vi "test_RS-xxx Protocol Factory.vi"(8 "error in (no error)":errorcluster, 11 "TestCase in":refnum<class "Instrument Addon Scripting API Protocol Factories Unit Tests.lvclass">) -> (0 "error out":errorcluster, 3 "TestCase out":refnum<class "Instrument Addon Scripting API Protocol Factories Unit Tests.lvclass">)   [LabVIEW 2018, in "Instrument Addon Scripting API Protocol Factories Unit Tests.lvclass"]
uses:
  Instrument Addon Scripting API Protocol Factories Unit Tests.lvclass
  RS-xxx/RS-xxx Settings.ctl
  RS-xxx/RS-xxx.lvclass
  RS-xxx/RS-xxx.lvclass/RS-xxx.ctl
  RS-xxx/Data Access/Read PortSettings.vi
  <vilib>/addons/_JKI Toolkits/VI Tester/TestCase.llb/TestCase.lvclass
  C:/Program Files (x86)/National Instruments/LabVIEW 2018/vi.lib/addons/_JKI Toolkits/VI Tester/TestCase.llb/TestCase.lvclass
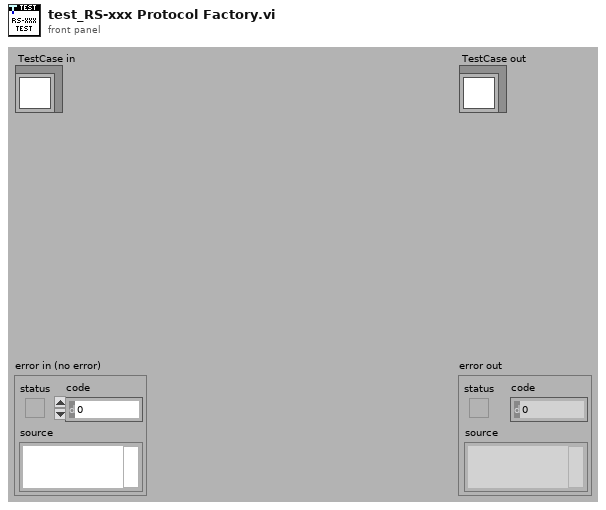
[diagram p1: front panel]
types:
  T1 = typedef "Protocols.lvlib/RS-xxx.lvclass/RS-xxx Settings.ctl" = cluster{"Port":string, "Baud Rate":u32, "Data Bits":u16, "Parity":enum16{"None", "Odd", "Even", "Mark", "Space"}, "Stop Bits":u16, "Flow Control":u16, "XON":enum16{"NUL", "SOH", "STX", "ETX", "EOT", "ENQ", "ACK", "BEL", "BS", "HT", "LF", "VT", "FF", "CR", "SO", "SI", "DLE", "DC1", "DC2", "DC3", "DC4", "NAK", "SYN", "ETB", "CAN", "EM", "SUB", "ESC", "FS", "GS", "RS", "US", "SP", "!", "\"", "#", "$", "%", "&", "'", "(", ")", "*", "+", ",", "- (-)", ".", "/", "0", "1", "2", "3", "4", "5", "6", "7", "8", "9", ":", ";", "<", "=", ">", "?", "@", "A", "B", "C", "D", "E", "F", "G", "H", "I", "J", "K", "L", "M", "N", "O", "P", "Q", "R", "S", "T", "U", "V", "W", "X", "Y", "Z", "[", "\\", "]", "^", "_", "`", "a", "b", "c", "d", "e", "f", "g", "h", "i", "j", "k", "l", "m", "n", "o", "p", "q", "r", "s", "t", "u", "v", "w", "x", "y", "z", "{", "|", "}", "~"}, "XOFF":enum16{"NUL", "SOH", "STX", "ETX", "EOT", "ENQ", "ACK", "BEL", "BS", "HT", "LF", "VT", "FF", "CR", "SO", "SI", "DLE", "DC1", "DC2", "DC3", "DC4", "NAK", "SYN", "ETB", "CAN", "EM", "SUB", "ESC", "FS", "GS", "RS", "US", "SP", "!", "\"", "#", "$", "%", "&", "'", "(", ")", "*", "+", ",", "- (-)", ".", "/", "0", "1", "2", "3", "4", "5", "6", "7", "8", "9", ":", ";", "<", "=", ">", "?", "@", "A", "B", "C", "D", "E", "F", "G", "H", "I", "J", "K", "L", "M", "N", "O", "P", "Q", "R", "S", "T", "U", "V", "W", "X", "Y", "Z", "[", "\\", "]", "^", "_", "`", "a", "b", "c", "d", "e", "f", "g", "h", "i", "j", "k", "l", "m", "n", "o", "p", "q", "r", "s", "t", "u", "v", "w", "x", "y", "z", "{", "|", "}", "~"}, "End Read on Termination Character":bool, "End Write on Termination Character":bool, "Termination Character":u8}
  T2 = cluster{"Port":string, "Baud Rate":u32, "Data Bits":u16, "Parity":enum16{"None", "Odd", "Even", "Mark", "Space"}, "Stop Bits":u16, "Flow Control":u16, "XON":enum16{"NUL", "SOH", "STX", "ETX", "EOT", "ENQ", "ACK", "BEL", "BS", "HT", "LF", "VT", "FF", "CR", "SO", "SI", "DLE", "DC1", "DC2", "DC3", "DC4", "NAK", "SYN", "ETB", "CAN", "EM", "SUB", "ESC", "FS", "GS", "RS", "US", "SP", "!", "\"", "#", "$", "%", "&", "'", "(", ")", "*", "+", ",", "- (-)", ".", "/", "0", "1", "2", "3", "4", "5", "6", "7", "8", "9", ":", ";", "<", "=", ">", "?", "@", "A", "B", "C", "D", "E", "F", "G", "H", "I", "J", "K", "L", "M", "N", "O", "P", "Q", "R", "S", "T", "U", "V", "W", "X", "Y", "Z", "[", "\\", "]", "^", "_", "`", "a", "b", "c", "d", "e", "f", "g", "h", "i", "j", "k", "l", "m", "n", "o", "p", "q", "r", "s", "t", "u", "v", "w", "x", "y", "z", "{", "|", "}", "~"}, "XOFF":enum16{"NUL", "SOH", "STX", "ETX", "EOT", "ENQ", "ACK", "BEL", "BS", "HT", "LF", "VT", "FF", "CR", "SO", "SI", "DLE", "DC1", "DC2", "DC3", "DC4", "NAK", "SYN", "ETB", "CAN", "EM", "SUB", "ESC", "FS", "GS", "RS", "US", "SP", "!", "\"", "#", "$", "%", "&", "'", "(", ")", "*", "+", ",", "- (-)", ".", "/", "0", "1", "2", "3", "4", "5", "6", "7", "8", "9", ":", ";", "<", "=", ">", "?", "@", "A", "B", "C", "D", "E", "F", "G", "H", "I", "J", "K", "L", "M", "N", "O", "P", "Q", "R", "S", "T", "U", "V", "W", "X", "Y", "Z", "[", "\\", "]", "^", "_", "`", "a", "b", "c", "d", "e", "f", "g", "h", "i", "j", "k", "l", "m", "n", "o", "p", "q", "r", "s", "t", "u", "v", "w", "x", "y", "z", "{", "|", "}", "~"}, "End Read on Termination Character":bool, "End Write on Termination Character":bool, "Termination Character":u8}
  T3 = enum16{"NUL", "SOH", "STX", "ETX", "EOT", "ENQ", "ACK", "BEL", "BS", "HT", "LF", "VT", "FF", "CR", "SO", "SI", "DLE", "DC1", "DC2", "DC3", "DC4", "NAK", "SYN", "ETB", "CAN", "EM", "SUB", "ESC", "FS", "GS", "RS", "US", "SP", "!", "\"", "#", "$", "%", "&", "'", "(", ")", "*", "+", ",", "- (-)", ".", "/", "0", "1", "2", "3", "4", "5", "6", "7", "8", "9", ":", ";", "<", "=", ">", "?", "@", "A", "B", "C", "D", "E", "F", "G", "H", "I", "J", "K", "L", "M", "N", "O", "P", "Q", "R", "S", "T", "U", "V", "W", "X", "Y", "Z", "[", "\\", "]", "^", "_", "`", "a", "b", "c", "d", "e", "f", "g", "h", "i", "j", "k", "l", "m", "n", "o", "p", "q", "r", "s", "t", "u", "v", "w", "x", "y", "z", "{", "|", "}", "~"}
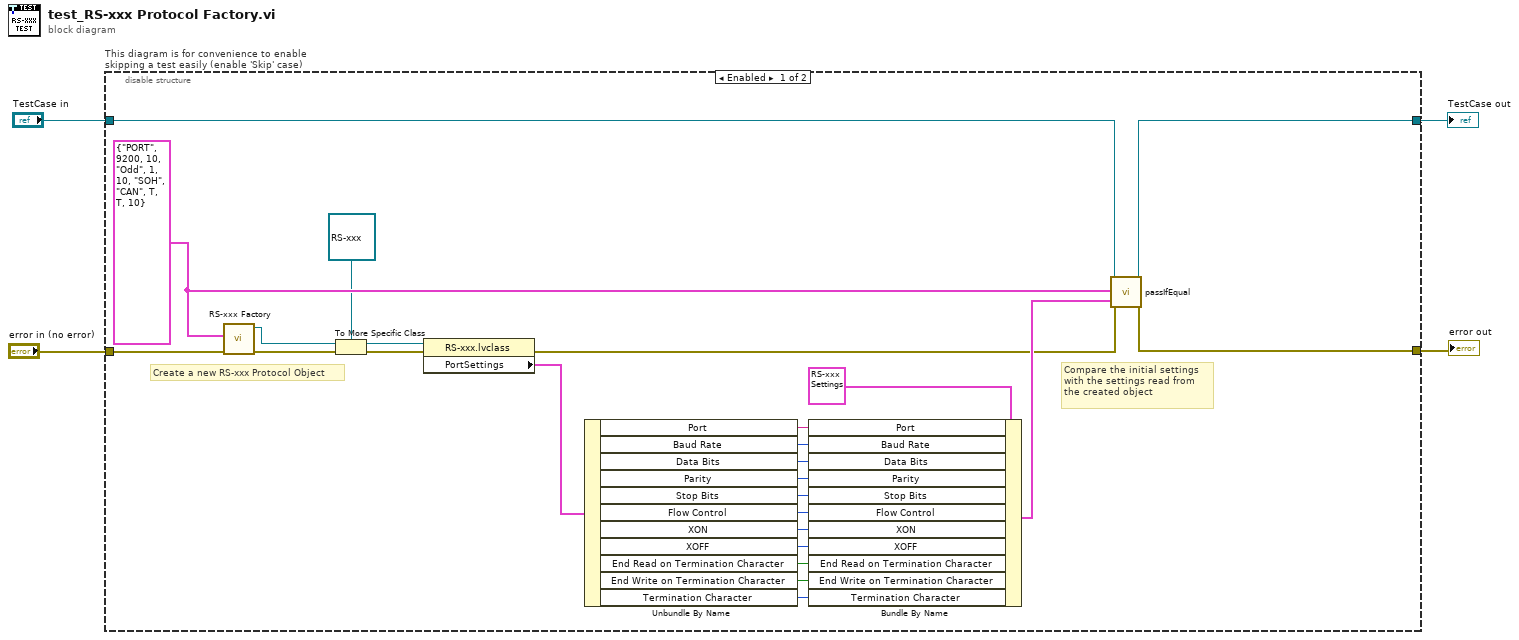
[diagram p0: block diagram]
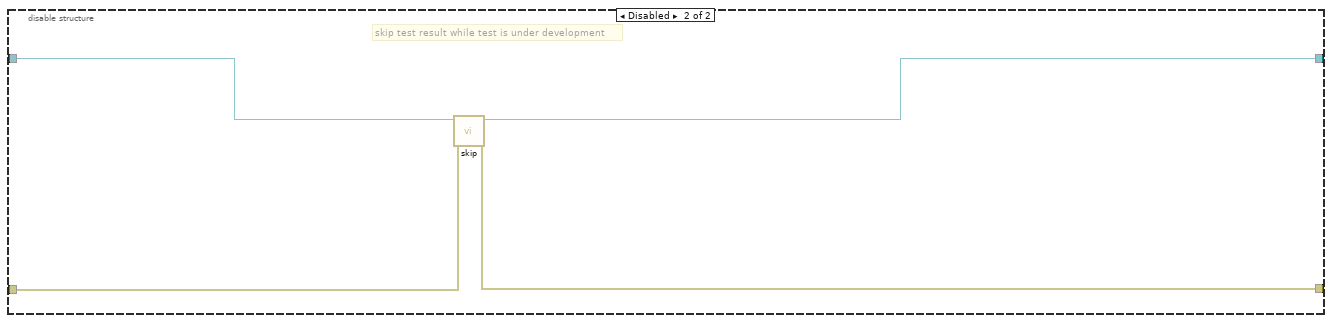
[diagram p2: hidden frame]
diagram:
  n1 = disable-structure "This diagram is for convenience to enable skipping a test easily (enable 'Skip' case)" shown="Enabled" {
    disable-tunnel: "TestCase in" -> [w29 w33]
    disable-tunnel: [w28 w31] -> w1
    disable-tunnel: [w27 w32] -> w3
    disable-tunnel: "error in (no error)" -> [w26 w30]
    frame Enabled {
      w23 = T1 {"Port"="PORT", "Baud Rate"=9200, "Data Bits"=10, "Parity"=enum."Odd", "Stop Bits"=1, "Flow Control"=10, "XON"=enum."SOH", "XOFF"=enum."CAN", "End Read on Termination Character"=TRUE, "End Write on Termination Character"=TRUE, "Termination Character"=10} ("Port Settings")
      # "Compare the initial settings \nwith the settings read from \nthe created object"
      # "Create a new RS-xxx Protocol Object"
      n2 = call "RS-xxx Factory.vi"("error in (no error)"=w26, "RS-xxx settings"=w23) -> ("error out"=w18:errorcluster, "protocol out"=w17:refnum<class "Protocol Parent.lvclass">)  [unwired: 8 in]
      n3 = To More Specific Class(target class=refnum<class "RS-xxx.lvclass"> refnum ("Protocols.lvlib:RS-xxx.lvclass"), reference=w17, error in=w18) -> (specific class reference=w20:refnum<class "RS-xxx.lvclass">, error out=w19:errorcluster)
      n4 = property class="RS-xxx.lvclass"(reference=w20, error in=w19) -> (error out=w22:errorcluster, "PortSettings"=w21:T2)  [unwired: 1 out]
      n5 = Unbundle By Name(w21) -> ("Port"=w15:string, "Baud Rate"=w14:u32, "Data Bits"=w13:u16, "Parity"=w12:enum16{"None", "Odd", "Even", "Mark", "Space"}, "Stop Bits"=w11:u16, "Flow Control"=w10:u16, "XON"=w9:T3, "XOFF"=w8:T3, "End Read on Termination Character"=w7:bool, "End Write on Termination Character"=w6:bool, "Termination Character"=w5:u8)
      n6 = Bundle By Name(cluster=T1 {"Port"="", "Baud Rate"=0, "Data Bits"=0, "Parity"=enum."None", "Stop Bits"=0, "Flow Control"=0, "XON"=enum."NUL", "XOFF"=enum."NUL", "End Read on Termination Character"=FALSE, "End Write on Termination Character"=FALSE, "Termination Character"=0} ("PortSettings"), "Port"=w15, "Baud Rate"=w14, "Data Bits"=w13, "Parity"=w12, "Stop Bits"=w11, "Flow Control"=w10, "XON"=w9, "XOFF"=w8, "End Read on Termination Character"=w7, "End Write on Termination Character"=w6, "Termination Character"=w5) -> (w24:T1)
      n7 = call-dynamic "passIfEqual.vi"("error in (no error)"=w22, "y"=w24, "x"=w23, "TestCase in"=w29) -> ("error out"=w27:errorcluster, "TestCase out"=w28:refnum<class "Instrument Addon Scripting API Protocol Factories Unit Tests.lvclass">)  [unwired: 6 in]
    }
    frame Disabled {
      # "skip test result while test is under development"
      n8 = call <vilib>:"skip.vi"("error in (no error)"=w30, "TestCase in"=w33) -> ("error out"=w32:errorcluster, "TestCase out"=w31:refnum<class "Instrument Addon Scripting API Protocol Factories Unit Tests.lvclass">)  [unwired: 8 in]
    }
  }
  "error out" <- w3
  "TestCase out" <- w1
